vi "Read_date_time_string.vi"(10 "Time":string, 11 "Date":string) -> (1 "Y/M/D/H/M/S":dbl[](array[numeric]), 2 "time in seconds":dbl format="%.2f", 3 "time stamp":timestamp, 5 "date time record":T1)   [LabVIEW 2012]
uses:
  <vilib>/Utility/miscctls.llb/LVDateTimeRec.ctl
panel:
  out "offset past match":i32
  out "hour":dbl
  out "minutes":dbl
  out "seconds":dbl
  out "Year":dbl
  out "day of month":dbl
  out "month":dbl
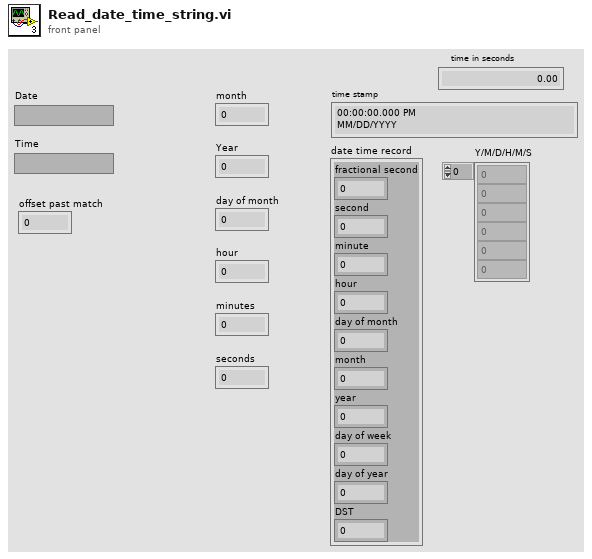
[diagram p1: front panel]
types:
  T1 = typedef "LVDateTimeRec.ctl" = cluster{"fractional second":dbl, "second":i32, "minute":i32, "hour":i32, "day of month":i32, "month":i32, "year":i32, "day of week":i32, "day of year":i32, "DST":i32}
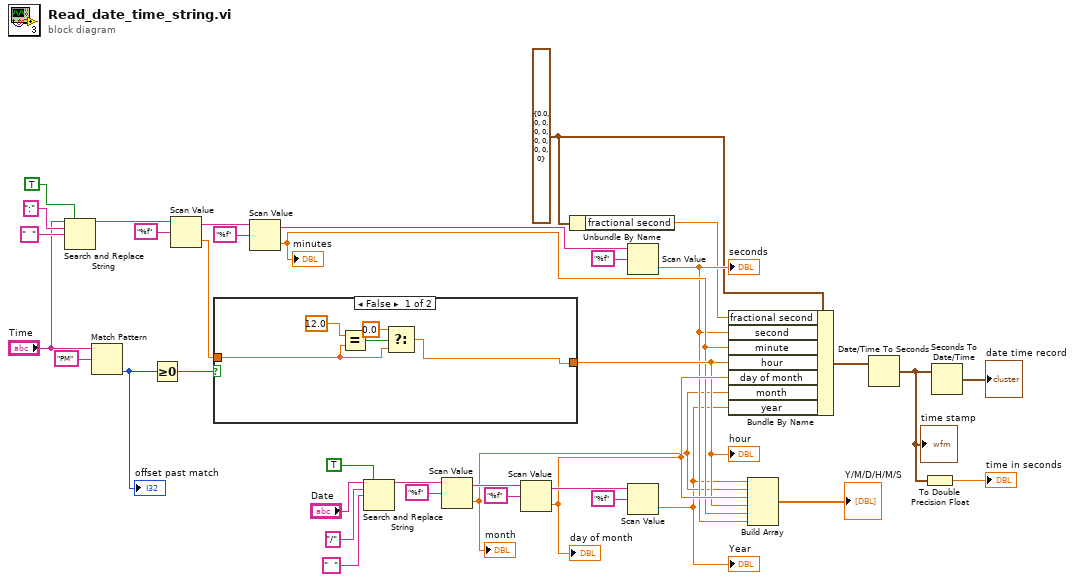
[diagram p0: block diagram]
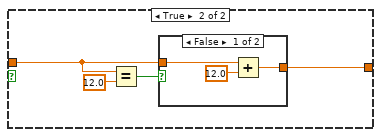
[diagram p2: hidden frame]
diagram:
  w5 = T1 {"fractional second"=0.0, "second"=0, "minute"=0, "hour"=0, "day of month"=0, "month"=0, "year"=0, "day of week"=0, "day of year"=0, "DST"=0}
  n1 = Search and Replace String(replace all?=TRUE ("replace all? (F)"), input string="Time", search string=":", replace string="  " ("replace string (\"\")")) -> (result string=w26:string)  [unwired: 4 in, 3 out]
  n2 = Match Pattern(string="Time", regular expression="PM") -> (offset past match=w18:i32)  [unwired: 1 in, 3 out]
  "offset past match" <- w18
  n3 = Greater Or Equal To 0?(x=w18) -> (x >= 0?=w17:bool)
  n4 = Scan Value(string=w26, format string="%f") -> (output string=w22:string, value=w16:dbl)  [unwired: 1 in]
  n5 = case shown="False" w17 {
    tunnel: w16 -> [w39 w44]
    tunnel: [w38 w46] -> w12
    frame False {
      n6 = Equal?(x=12.0 ("y"), y=w39) -> (x = y?=w42:bool)
      n7 = Select(t=0.0, s=w42, f=w39) -> (s? t:f=w38:dbl)
    }
    frame True {
      n8 = Equal?(x=w44, y=12.0) -> (x = y?=w45:bool)
      n9 = case shown="False" w45 {
        tunnel: w44 -> [w49 w50]
        tunnel: [w47 w50] -> w46
        frame False {
          n10 = Add(x=w49, y=12.0) -> (x+y=w47:dbl)
        }
        frame True {
        }
      }
    }
  }
  "hour" <- w12
  n11 = Scan Value(string=w22, format string="%f") -> (output string=w28:string, value=w11:dbl)  [unwired: 1 in]
  "minutes" <- w11
  n12 = Search and Replace String(replace all?=TRUE ("replace all? (F)"), input string="Date", search string="/", replace string="  " ("replace string (\"\")")) -> (result string=w31:string)  [unwired: 4 in, 3 out]
  n13 = Scan Value(string=w31, format string="%f") -> (output string=w35:string, value=w7:dbl)  [unwired: 1 in]
  "month" <- w7
  n14 = Scan Value(string=w35, format string="%f") -> (output string=w29:string, value=w13:dbl)  [unwired: 1 in]
  "day of month" <- w13
  n15 = Unbundle By Name(w5) -> ("fractional second"=w8:dbl)
  n16 = Scan Value(string=w28, format string="%f") -> (value=w10:dbl)  [unwired: 1 in, 1 out]
  "seconds" <- w10
  n17 = Scan Value(string=w29, format string="%f") -> (value=w6:dbl)  [unwired: 1 in, 1 out]
  "Year" <- w6
  n18 = Bundle By Name(cluster=w5, "fractional second"=w8, "second"=w10, "minute"=w11, "hour"=w12, "day of month"=w13, "month"=w7, "year"=w6) -> (w4:T1)
  n19 = Build Array(w6, w7, w13, w12, w11, w10) -> (→"Y/M/D/H/M/S":dbl[])
  n20 = Date/Time To Seconds(2:w4) -> (0:w2:timestamp)  [unwired: 1 in]
  "time stamp" <- w2
  n21 = To Double Precision Float(number=w2) -> (double precision float=→"time in seconds":dbl)
  n22 = Seconds To Date/Time(time stamp (now)=w2) -> (date time rec=→"date time record":T1)  [unwired: 1 in]
